vi "XY Graph Show-Hide Tool Panels Event.vi"(8 "Error In":errorcluster, 11 "XYGraph in":T1) -> (0 "Error Out":errorcluster, 1 "Message":string)   [LabVIEW 2019, in "XY Graph Add-Ons.lvlib"]
uses:
  XY Graph Add-Ons.lvlib
  XY Graph Refnum.ctl
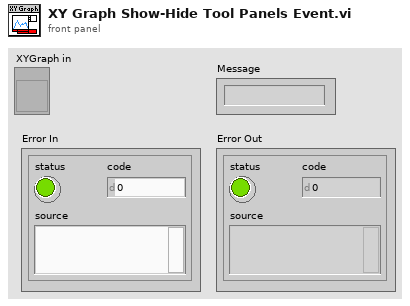
[diagram p1: front panel]
types:
  T1 = typedef "XY Graph Add-Ons.lvlib/XY Graph Refnum.ctl" = refnum<vi>
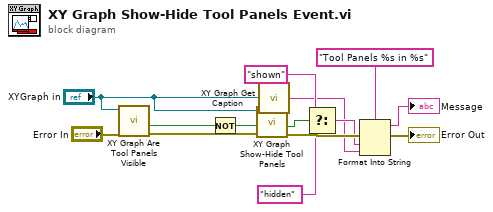
[diagram p0: block diagram]
diagram:
  n1 = call "XY Graph Are Tool Panels Visible.vi"("Error In"="Error In", "XY Graph Ref"="XYGraph in") -> ("Error Out"=w3:errorcluster, "Any Panel Visible?"=w2:bool)  [unwired: 7 in, 1 out]
  n2 = Not(x=w2) -> (.not. x?=w1:bool)
  n3 = call "XY Graph Show-Hide Tool Panels.vi"("Error In"=w3, "Hide (F) /Show (T)"=w1, "XY Graph Ref"="XYGraph in") -> ("Error Out"=w14:errorcluster, "Tool Panels Shown?"=w10:bool)  [unwired: 7 in]
  n4 = call "XY Graph Get Caption.vi"("XYGraph"="XYGraph in") -> ("Graph Caption"=w6:string)  [unwired: 8 in]
  n5 = Select(t="shown" ("format string"), s=w10, f="hidden" ("format string")) -> (s? t:f=w7:string)
  n6 = Format Into String(format string="Tool Panels %s in %s", error in=w14, w7, w6) -> (resulting string=→"Message":string, error out=→"Error Out":errorcluster)  [unwired: 1 in]
